vi "Tester_Create.vi"(8 "Error In":errorcluster, 10 "Mediator":refnum<class "Mediator.lvclass">, 11 "reference in":refnum<class "Tester.lvclass">) -> (0 "Error Out":errorcluster, 3 "reference out":refnum<class "Tester.lvclass">)   [LabVIEW 2020, in "Tester.lvclass"]
uses:
  Tester.lvclass
  C:/Projects/DesignPatterns/Mediator/Colleague_class/Colleague.lvclass
  Mediator_class/Mediator.lvclass
  Colleague_class/Colleague.lvclass
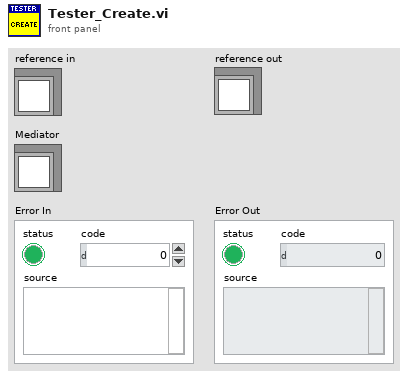
[diagram p1: front panel]
types:
  T1 = typedef "Tester.lvclass/ObjectAttributes.ctl" = cluster{"None":bool}
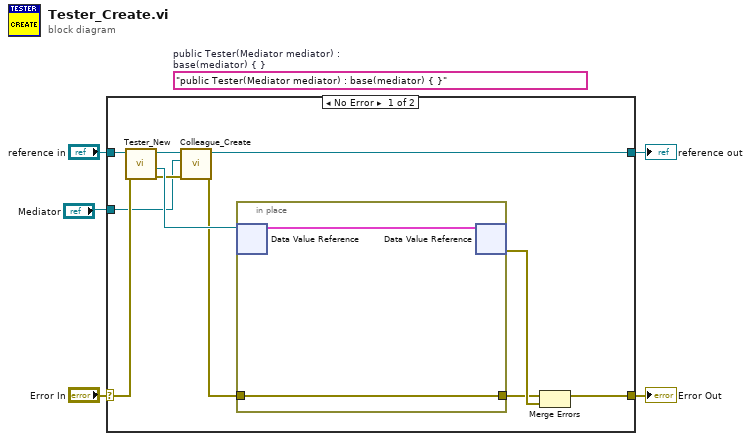
[diagram p0: block diagram]
diagram:
  (unwired) "public Tester(Mediator mediator) : base(mediator) { }"  # public Tester(Mediator mediator) : base(mediator) { }
  n1 = case shown="No Error" "Error In" {
    selector: "Error In" -> [w12 w20]
    tunnel: [w10 w20] -> w4
    tunnel: "reference in" -> [w14 w19]
    tunnel: [w9 w19] -> w2
    tunnel: "Mediator" -> [w6 _]
    frame No Error {
      n2 = call "Tester_New.vi"("error in (no error)"=w12, "reference in"=w14) -> ("error out"=w13:errorcluster, "DVRRefOut"=w16:refnum<data-value>, "reference out"=w15:refnum<class "Tester.lvclass">)  [unwired: 6 in, 1 out]
      n3 = call "Colleague_Create.vi"("Error In"=w13, "Mediator"=w6, "reference in"=w15) -> ("Error Out"=w8:errorcluster, "reference out"=w9:refnum<class "Tester.lvclass">)  [unwired: 7 in]
      n4 = in-place {
        in-place-border: w8 -> [w18]
        in-place-border: [w18] -> w7
        n5 = in-place-dvr #1(w16) -> (w17:T1)  [unwired: 1 out]
        n6 = in-place-dvr #1(w17) -> (w11:errorcluster)  [unwired: 1 out]
      }
      n7 = Merge Errors(w7, w11) -> (w10:errorcluster)
    }
    frame Error {
    }
  }
  "Error Out" <- w4
  "reference out" <- w2
